vi "Binary String to Decimal Number_LV2012_NI Verified.vi"(9 "String":string="101") -> (1 "Number":u64)   [LabVIEW 2017]
doc: "This VI allows to convert a binary String into the correct numeric representation"
panel:
  # "Overview: This VI allows you to convert a binary String into the correct numeric representation\nRequirements: LabVIEW 2012(or compatible)\nInstructions:\n1. Enter the binary number\n2. Run the VI"
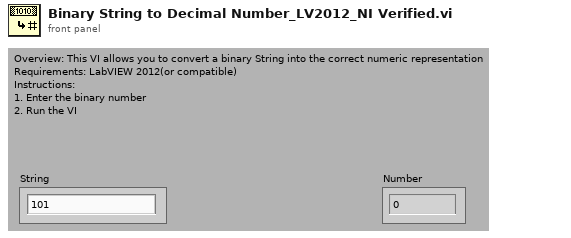
[diagram p1: front panel]
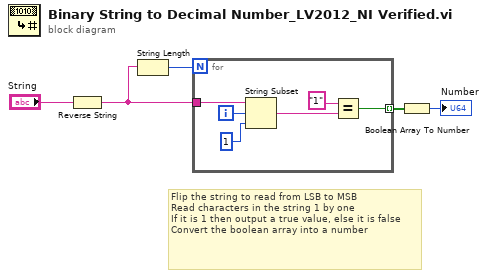
[diagram p0: block diagram]
diagram:
  # "Flip the string to read from LSB to MSB\nRead characters in the string 1 by one\nIf it is 1 then output a true value, else it is false\nConvert the boolean array into a number"
  n1 = Reverse String(1:"String") -> (0:w2:string)
  n2 = String Length(string=w2) -> (length=w5:i32)
  n3 = for {
    N: w5 -> [_]
    tunnel: w2 -> [w11]
    tunnel: [w6] -> w4 mode=indexing
    i -> [w9]
    n4 = String Subset(string=w11, offset (0)=w9, length (rest)=1 ("length (rest)")) -> (substring=w7:string)
    n5 = Equal?(x="1", y=w7) -> (x = y?=w6:bool)
  }
  n6 = Boolean Array To Number(Boolean array=w4) -> (number=→"Number":u32)
